vi "CCAR InsertProcess.vi"() -> ()   [LabVIEW 2022 SP3]
panel:
  out "ReplyTracMex":string
  in  "Employee":string
  in  "FailString":string
  in  "PassFail":i32
  in  "SerialNumber":string
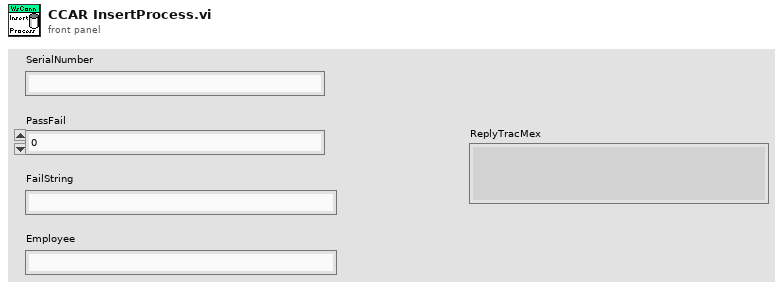
[diagram p1: front panel]
types:
  T1 = enum16{"Start Up", "RFID", "Power Display", "Internal Speaker", "Acceletometer", "Signal Network", "ALS", "Touch Display"}
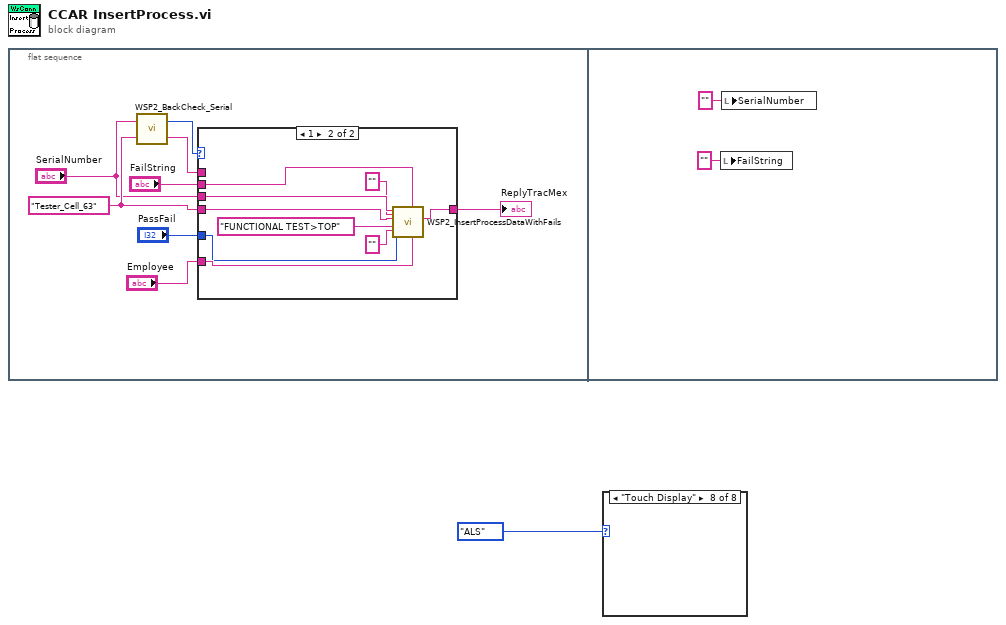
[diagram p0: block diagram]
diagram:
  n1 = flat-sequence {
    frame #0 {
      w9 = "Tester_Cell_63"
      n2 = call "WSP2_BackCheck_Serial.vi"("stationName"=w9, "serialNumber"="SerialNumber") -> ("ReplyTracMex"=w6:string, "Status"=w7:i8)
      n3 = case shown="1" w7 {
        tunnel: "SerialNumber" -> [_ w19]
        tunnel: w9 -> [_ w18]
        tunnel: w6 -> [w10 _]
        tunnel: [w10 w17] -> w5
        tunnel: "Employee" -> [_ w15]
        tunnel: "PassFail" -> [_ w14]
        tunnel: "FailString" -> [_ w12]
        frame 0, Default {
        }
        frame 1 {
          n4 = call "WSP2_InsertProcessDataWithFails.vi"("Employee"=w15, "FailString"=w12, "EndTime"="", "EntryTime"="", "PassFail"=w14, "ProcessName"="FUNCTIONAL TEST>TOP", "StationName"=w18, "SerialNumber"=w19) -> ("ReplyTrace"=w17:string)  [unwired: 3 in]
        }
      }
      "ReplyTracMex" <- w5
    }
    frame #1 {
      n5 = local write "FailString"("" ("FailString")) -> ()
      n6 = local write "SerialNumber"("" ("SerialNumber")) -> ()
    }
  }
  n7 = case shown="\"Touch Display\"" T1."ALS" {
    frame "Start Up", Default {
    }
    frame "RFID" {
    }
    frame "Power Display" {
    }
    frame "Internal Speaker" {
    }
    frame "Acceletometer" {
    }
    frame "Signal Network" {
    }
    frame "ALS" {
    }
    frame "Touch Display" {
    }
  }
